vi "TESTER.vi"() -> ()   [LabVIEW 2011]
panel:
  in  "Write Temperature":dbl=25.0
  in  "Bypass Ducat AutoSearch":bool
  in  "Ducat":string="ducat3"
  in  "SRP Server Name":string="jit3"
  in  "stop":bool
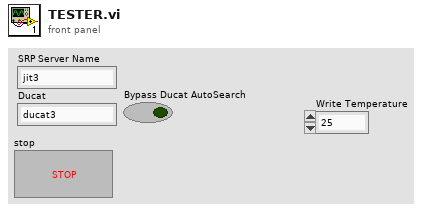
[diagram p1: front panel]
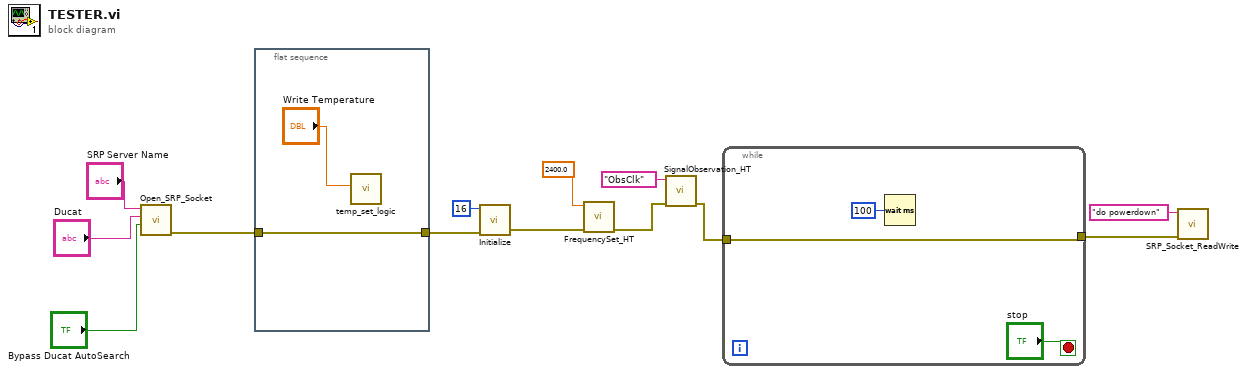
[diagram p0: block diagram]
diagram:
  n1 = call "Open_SRP_Socket.vi"("Bypass Ducat AutoSearch"="Bypass Ducat AutoSearch", "Ducat Name"="Ducat", "SRP Server Name"="SRP Server Name") -> ("error out"=w10:errorcluster)  [unwired: 6 in, 2 out]
  n2 = flat-sequence {
    tunnel: w10 -> [w14]
    tunnel: [w14] -> w8
    frame #0 {
      n3 = call "temp_set_logic.vi"("Write Temperature"="Write Temperature") -> ()  [unwired: 10 in, 1 out]
    }
  }
  n4 = call "Initialize.vi"("error in"=w8, "RegRefAdj"=16) -> ("error out"=w6:errorcluster)  [unwired: 7 in]
  n5 = call "FrequencySet_HT.vi"("error in"=w6, "VCO Frequency"=2400.0 ("NB VCO Frequency")) -> ("error out"=w4:errorcluster)  [unwired: 7 in]
  n6 = call "SignalObservation_HT.vi"("error in (no error)"=w4, "Signal"="ObsClk") -> ("error out"=w1:errorcluster)  [unwired: 7 in]
  n7 = while {
    tunnel: [w16] -> w2
    tunnel: w1 -> [w16]
    stop <- "stop" stop-if-true
    n8 = Wait (ms)(milliseconds to wait=u32 100) -> ()  [unwired: 1 out]
  }
  n9 = call "SRP_Socket_ReadWrite.vi"("error in (no error)"=w2, "Data In"="do powerdown") -> ()  [unwired: 7 in, 2 out]
